vi "WS1021 Individual Beam Controls.vi"(8 "Error In":errorcluster, 11 "USID":string="07") -> (0 "Error Out":errorcluster, 1 "Reg 2 Cmd":string[](array[string]), 2 "Reg 3 Cmd":string[](array[string]), 3 "Reg 2 Name":string[](array[string]), 4 "VPI_Cmd":string[](array[string])=["07437F", "074300", "07427F", "074200"], 5 "Reg 3 Name":string[](array[string]), 7 "VPI_Name":string[](array[string])=["07437F", "074300", "07427F", "074200"])   [LabVIEW 2017]
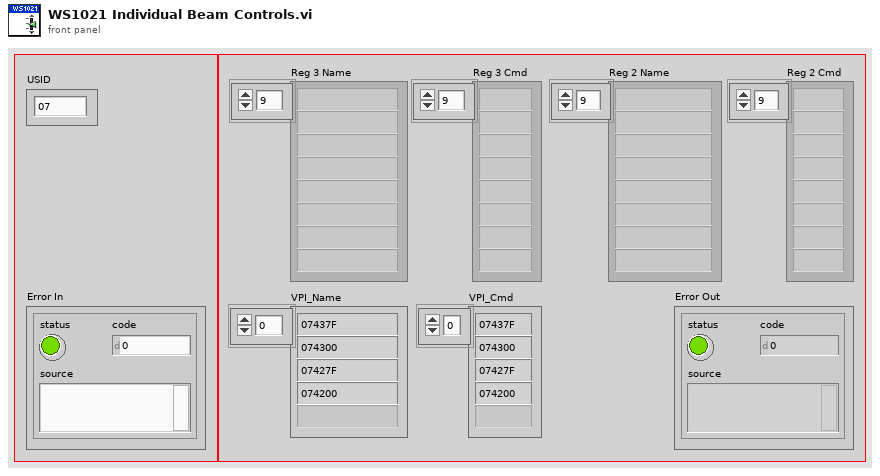
[diagram p1: front panel]
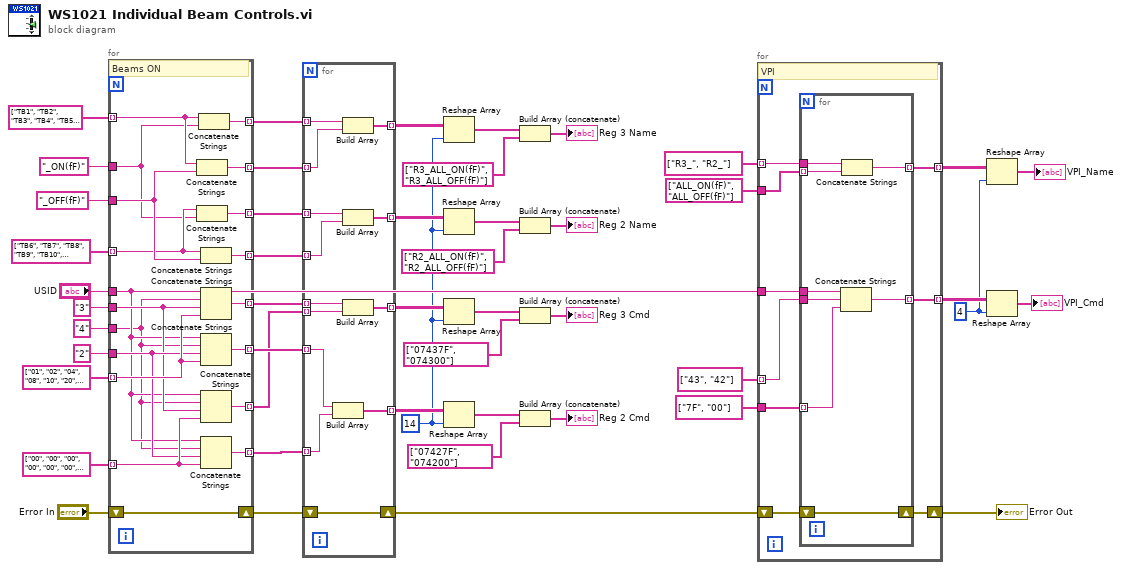
[diagram p0: block diagram]
diagram:
  w13 = 14 ("dimension size")
  w32 = 4 ("dimension size")
  n1 = for {
    tunnel: string[] ["TB1", "TB2", "TB3", "TB4", "TB5", "FB3", "FB1"] ("Reg 3 Name") -> [w54] mode=indexing
    tunnel: string[] ["TB6", "TB7", "TB8", "TB9", "TB10", "TB11", "FB2"] ("Reg 2 Name") -> [w50] mode=indexing
    tunnel: [w64] -> w27 mode=indexing
    tunnel: [w63] -> w26 mode=indexing
    tunnel: string[] ["01", "02", "04", "08", "10", "20", "40"] ("8 Bits") -> [w65] mode=indexing
    tunnel: "USID" -> [w58]
    tunnel: "4" ("R/W Cmd") -> [w57]
    tunnel: [w67] -> w25 mode=indexing
    tunnel: [w62] -> w24 mode=indexing
    shift-right: [w66] -> w29
    shift-left: "Error In" -> [w66]
    tunnel: "3" ("Reg 3") -> [w59]
    tunnel: "2" ("Reg 2") -> [w60]
    tunnel: "_ON(fF)" -> [w49]
    tunnel: string[] ["00", "00", "00", "00", "00", "00", "00"] ("8 Bits") -> [w61] mode=indexing
    tunnel: [w56] -> w22 mode=indexing
    tunnel: [w55] -> w21 mode=indexing
    tunnel: "_OFF(fF)" -> [w51]
    tunnel: [w53] -> w18 mode=indexing
    tunnel: [w52] -> w19 mode=indexing
    # "Beams ON"
    n2 = Concatenate Strings(w54, w51) -> (w53:string)
    n3 = Concatenate Strings(w50, w49) -> (w52:string)
    n4 = Concatenate Strings(w54, w49) -> (w64:string)
    n5 = Concatenate Strings(w50, w51) -> (w63:string)
    n6 = Concatenate Strings(w58, w57, w59, w65) -> (w67:string)
    n7 = Concatenate Strings(w58, w57, w60, w65) -> (w62:string)
    n8 = Concatenate Strings(w58, w57, w59, w61) -> (w56:string)
    n9 = Concatenate Strings(w58, w57, w60, w61) -> (w55:string)
  }
  n10 = for {
    shift-right: [w80] -> w28
    shift-left: w29 -> [w80]
    tunnel: w27 -> [w75] mode=indexing
    tunnel: w26 -> [w72] mode=indexing
    tunnel: w25 -> [w78] mode=indexing
    tunnel: w24 -> [w79] mode=indexing
    tunnel: w22 -> [w77] mode=indexing
    tunnel: w21 -> [w76] mode=indexing
    tunnel: w19 -> [w73] mode=indexing
    tunnel: w18 -> [w74] mode=indexing
    tunnel: [w71] -> w17 mode=indexing
    tunnel: [w70] -> w16 mode=indexing
    tunnel: [w69] -> w15 mode=indexing
    tunnel: [w68] -> w14 mode=indexing
    n11 = Build Array(w79, w76) -> (w71:string[])
    n12 = Build Array(w75, w74) -> (w69:string[])
    n13 = Build Array(w73, w72) -> (w68:string[])
    n14 = Build Array(w78, w77) -> (w70:string[])
  }
  n15 = Reshape Array(w15, w13) -> (w12:string[])
  n16 = Reshape Array(w14, w13) -> (w9:string[])
  n17 = Reshape Array(w16, w13) -> (w5:string[])
  n18 = Reshape Array(w17, w13) -> (w3:string[])
  n19 = Build Array (concatenate)(w12, string[] ["R3_ALL_ON(fF)", "R3_ALL_OFF(fF)"]) -> (→"Reg 3 Name":string[])
  n20 = Build Array (concatenate)(w9, string[] ["R2_ALL_ON(fF)", "R2_ALL_OFF(fF)"]) -> (→"Reg 2 Name":string[])
  n21 = Build Array (concatenate)(w5, string[] ["07437F", "074300"]) -> (→"Reg 3 Cmd":string[])
  n22 = Build Array (concatenate)(w3, string[] ["07427F", "074200"]) -> (→"Reg 2 Cmd":string[])
  n23 = for {
    tunnel: string[] ["R3_", "R2_"] ("VPI_Name") -> [w88] mode=indexing
    tunnel: string[] ["ALL_ON(fF)", "ALL_OFF(fF)"] -> [w89]
    tunnel: string[] ["7F", "00"] -> [w85]
    tunnel: "USID" -> [w87]
    tunnel: string[] ["43", "42"] -> [w86] mode=indexing
    tunnel: [w84] -> w34 mode=indexing
    tunnel: [w83] -> w36 mode=indexing
    shift-right: [w81] -> w31
    shift-left: w28 -> [w82]
    # "VPI"
    n24 = for {
      tunnel: w89 -> [w97] mode=indexing
      tunnel: w88 -> [w96]
      tunnel: [w95] -> w83 mode=indexing
      tunnel: w87 -> [w94]
      tunnel: w86 -> [w93]
      tunnel: w85 -> [w92] mode=indexing
      tunnel: [w91] -> w84 mode=indexing
      shift-right: [w90] -> w81
      shift-left: w82 -> [w90]
      n25 = Concatenate Strings(w94, w93, w92) -> (w91:string)
      n26 = Concatenate Strings(w96, w97) -> (w95:string)
    }
  }
  "Error Out" <- w31
  n27 = Reshape Array(w36, w32) -> (→"VPI_Name":string[])
  n28 = Reshape Array(w34, w32) -> (→"VPI_Cmd":string[])
